vi "Init Panels.vi"(8 "error in (no error)":errorcluster, 11 "picoG in":refnum<class "picoG.lvclass">) -> (0 "error out":errorcluster, 3 "picoG out":refnum<class "picoG.lvclass">)   [LabVIEW 2020, in "PicoG-App.lvlib" / "picoG.lvclass"]
uses:
  picoG.lvclass
  picoG.lvclass/picoG.ctl
  <vilib>/IlluminatedG/IG OOPanel/OOPanel/Manager/Manager.lvclass
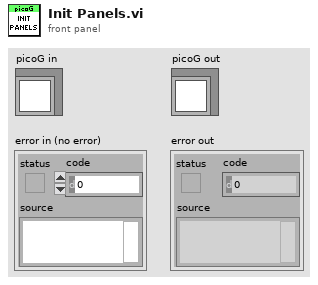
[diagram p1: front panel]
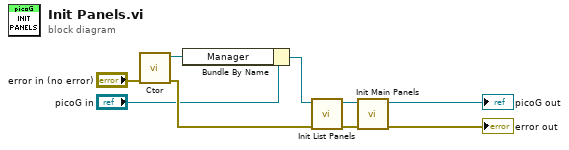
[diagram p0: block diagram]
diagram:
  n1 = call <vilib>:"Ctor.vi"("error in (no error)"="error in (no error)") -> ("error out"=w9:errorcluster, "Manager out"=w7:refnum<class "Manager.lvclass">)  [unwired: 9 in]
  n2 = Bundle By Name(cluster="picoG in", "Manager"=w7) -> (w2:refnum<class "picoG.lvclass">)
  n3 = call "Init List Panels.vi"("error in (no error)"=w9, "picoG in"=w2) -> ("error out"=w6:errorcluster, "picoG out"=w3:refnum<class "picoG.lvclass">)  [unwired: 8 in]
  n4 = call "Init Main Panels.vi"("error in (no error)"=w6, "picoG in"=w3) -> ("error out"=→"error out":errorcluster, "picoG out"=→"picoG out":refnum<class "picoG.lvclass">)  [unwired: 8 in]
